vi "NP_Logging.vi"(0 "Instrument Channel":string="GPIB/0:4,0", 1 "Prefix (Instrument name)":string, 2 "String 1 Enable (T)":bool=TRUE, 3 "Generic Strings":bool, 5 "String 1 {Write} (in)":string, 7 "String 2 {Read} (in)":string, 9 "Filename (Data.log)":string="Data.log", 11 "error in (no error)":errorcluster, 12 "Operating Mode (Logging)":T1=enum."Logging", 13 "String 2 Enable (T)":bool=TRUE) -> (4 "Instrument Channel out":string="GPIB/0:4,0", 6 "String 1 {Write} (out)":string, 8 "String 2 {Read} (out)":string, 15 "error out":errorcluster)   [LabVIEW 2013]
doc: "This VI will enable logging of communication to a text file.\n\nIt will put timestamp and strings in the log file. \n\nIt can be used for Query/Response, or Generically for any logging.\nThe Label will be after the timestamp.\n\nNormal Operating Mode will disable logging."
uses:
  ctl_OperatingMode.ctl
panel:
  out "Target path":path
  in  "Show Interval":bool
  # "If Generic then Prefix will not indicate Write and Response."
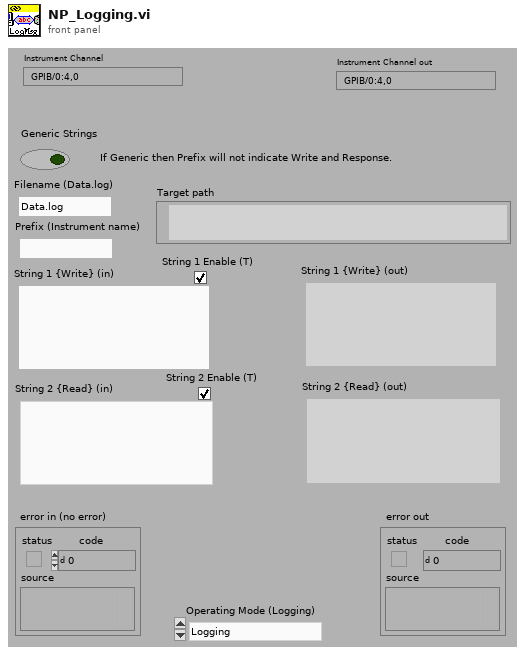
[diagram p1: front panel]
types:
  T1 = typedef "ctl_OperatingMode.ctl" = enum16{"Normal", "Logging", "Simulation w/Zeroes", "Simulation from Log File"}
  T2 = enum32{"invalid app kind", "Development System", "Run Time System", "Student Edition", "Embedded LabVIEW", "Evaluation", "Custom"}
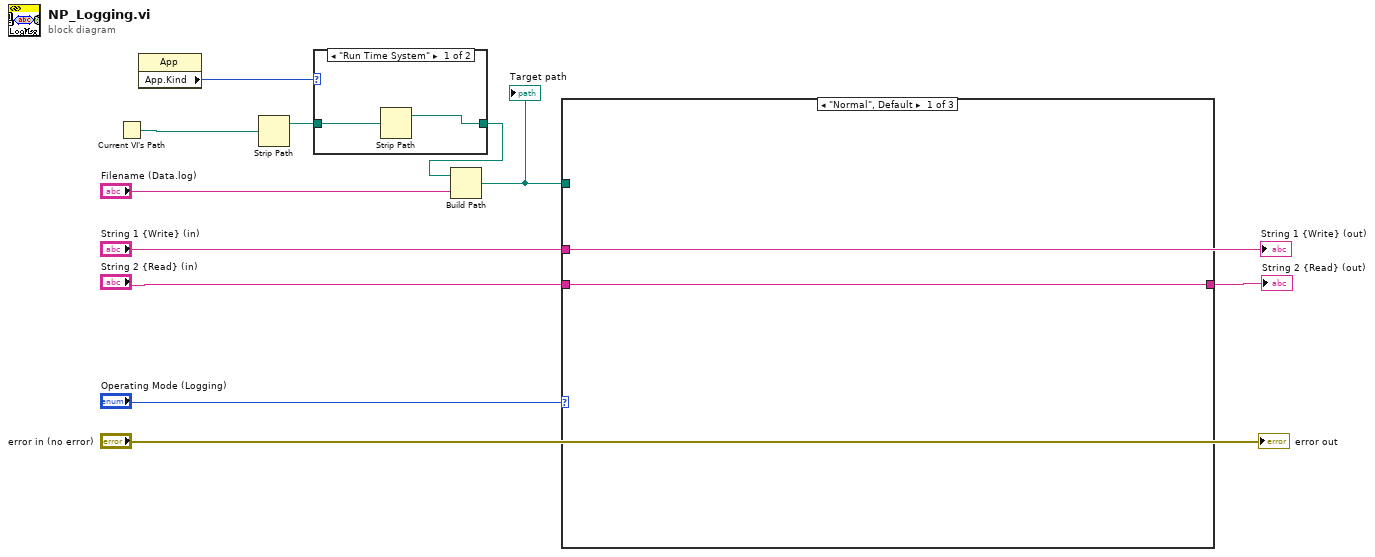
[diagram p0: block diagram]
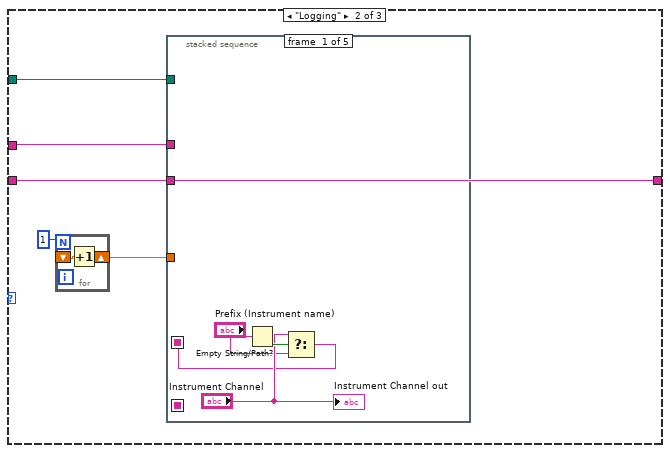
[diagram p3: hidden frame]
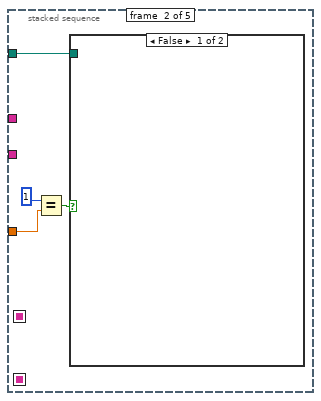
[diagram p4: hidden frame]
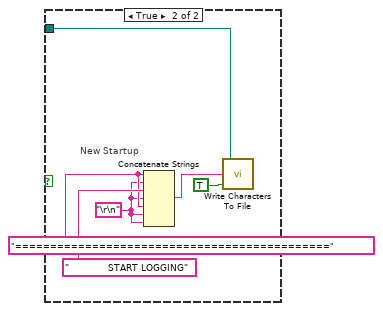
[diagram p5: hidden frame]
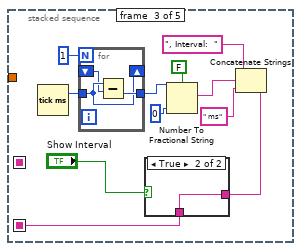
[diagram p6: hidden frame]
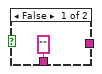
[diagram p7: hidden frame]
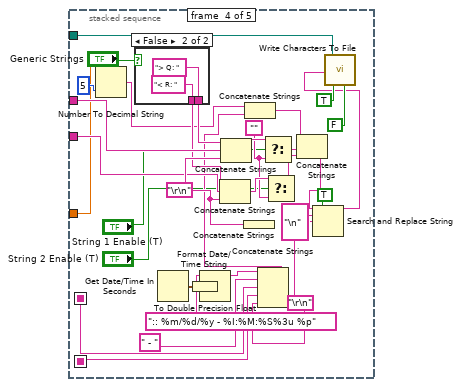
[diagram p8: hidden frame]
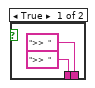
[diagram p9: hidden frame]
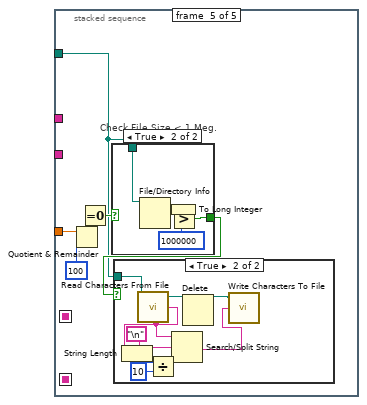
[diagram p10: hidden frame]
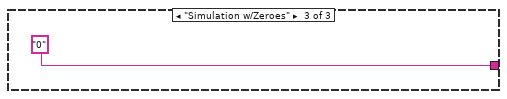
[diagram p13: hidden frame]
diagram:
  n1 = Current VI's Path() -> (path=w2:path)
  n2 = property class="App"() -> ("App.Kind"=w4:T2)  [unwired: 2 in, 2 out]
  n3 = Strip Path(path=w2) -> (stripped path=w3:path)  [unwired: 1 out]
  n4 = case shown="\"Run Time System\"" w4 {
    tunnel: w3 -> [w13 w14]
    tunnel: [w12 w14] -> w1
    frame "Run Time System" {
      n5 = Strip Path(path=w13) -> (stripped path=w12:path)  [unwired: 1 out]
    }
    frame Default {
    }
  }
  n6 = Build Path(base path=w1, name or relative path="Filename (Data.log)") -> (appended path=w5:path)
  "Target path" <- w5
  n7 = case shown="\"Normal\", Default" "Operating Mode (Logging)" {
    tunnel: "String 1 {Write} (in)" -> [_ w19 _]
    tunnel: "String 2 {Read} (in)" -> [w15 w20 _]
    tunnel: [w15 w20 "0"] -> w10
    tunnel: w5 -> [_ w18 _]
    frame "Normal", Default {
    }
    frame "Logging" {
      n8 = for {
        N: 1 -> [_]
        shift-right: [w21] -> w17
        shift-left: _ -> [w22]
        n9 = Increment(x=w22) -> (x+1=w21:dbl)
      }
      n10 = stacked-sequence {
        seq-local: [w23 _ _ _ _] -> [_ _ _ w62 _]
        seq-local: [_ _ w37 _ _] -> [_ _ _ w57 _]
        tunnel: w20 -> [_ _ _ w76 _]
        tunnel: w19 -> [_ _ _ w83 _]
        tunnel: w18 -> [_ w28 _ w54 w91]
        tunnel: w17 -> [_ w27 _ w53 w90]
        frame #0 {
          n11 = Empty String/Path?(string/path="Prefix (Instrument name)") -> (empty?=w26:bool)
          n12 = Select(t="Instrument Channel", s=w26, f="Prefix (Instrument name)") -> (s? t:f=w23:string)
          "Instrument Channel out" <- "Instrument Channel"
        }
        frame #1 {
          n13 = Equal?(x=1, y=w27) -> (x = y?=w29:bool)
          n14 = case shown="False" w29 {
            tunnel: w28 -> [_ w31]
            frame False {
            }
            frame True {
              w33 = "\r\n"
              w34 = "============================================="
              # "New Startup"
              n15 = Concatenate Strings(w34, w33, "             START LOGGING", w33, w34, w33, w33) -> (w32:string)
              n16 = call <vilib>:"Write Characters To File.vi"("append to file? (new file:F)"=TRUE, "character string"=w32, "file path (dialog if empty)"=w31) -> ()  [unwired: 2 in, 1 out]
            }
          }
        }
        frame #2 {
          n17 = Tick Count (ms)() -> (millisecond timer value=w47:u32)
          n18 = for {
            N: 1 -> [_]
            shift-right: [w51] -> _
            shift-left: _ -> [w50]
            tunnel: w47 -> [w51]
            tunnel: [w52] -> w45
            n19 = Subtract(x=w51, y=w50) -> (x-y=w52:u32)
          }
          n20 = Number To Fractional String(use system decimal point (T)=FALSE, number=w45, precision (6)=i16 0) -> (F-format string=w42:string)  [unwired: 1 in]
          n21 = Concatenate Strings(", Interval:  ", w42, " ms") -> (w38:string)
          n22 = case shown="True" "Show Interval" {
            tunnel: w38 -> [_ w49]
            tunnel: ["" w49] -> w37
            frame False {
            }
            frame True {
            }
          }
        }
        frame #3 {
          w67 = ""
          w77 = "\r\n"
          w56 = "\r\n"
          n23 = Number To Decimal String(number=w53, width (-)=i16 5) -> (decimal integer string=w74:string)
          n24 = case shown="False" "Generic Strings" {
            tunnel: [">>  " "< R: "] -> w75
            tunnel: [">>  " "> Q: "] -> w79
            frame True {
            }
            frame False {
            }
          }
          n25 = Get Date/Time In Seconds() -> (seconds since 1Jan1904=w55:timestamp)
          n26 = To Double Precision Float(number=w55) -> (double precision float=w82:dbl)
          n27 = Format Date/Time String(time format string (%c)=":: %m/%d/%y - %I:%M:%S%3u %p", seconds (now)=w82) -> (date/time string=w64:string)  [unwired: 1 in]
          n28 = Concatenate Strings(w75, w76, w77) -> (w71:string)
          n29 = Concatenate Strings(w79, w83, w77) -> (w69:string)
          n30 = Concatenate Strings(w77) -> ()  [unwired: 1 out]
          n31 = Concatenate Strings(w64, " - ", w62, w57, w56) -> (w73:string)
          n32 = Concatenate Strings(w74, w73) -> (w72:string)
          n33 = Select(t=w69, s="String 1 Enable (T)", f=w67) -> (s? t:f=w70:string)
          n34 = Select(t=w71, s="String 2 Enable (T)", f=w67) -> (s? t:f=w68:string)
          n35 = Concatenate Strings(w72, w70, w68) -> (w61:string)
          n36 = Search and Replace String(replace all?=TRUE ("replace all? (F)"), input string=w61, search string="\n", replace string=w56) -> (result string=w58:string)  [unwired: 4 in, 3 out]
          n37 = call <vilib>:"Write Characters To File.vi"("convert eol? (no:F)"=FALSE, "append to file? (new file:F)"=TRUE, "character string"=w58, "file path (dialog if empty)"=w54) -> ()  [unwired: 1 in, 1 out]
        }
        frame #4 {
          # "Check File Size < 1 Meg."
          n38 = Quotient & Remainder(x=w90, y=100) -> (x-y*floor(x/y)=w94:i32)  [unwired: 1 out]
          n39 = Equal To 0?(x=w94) -> (x = 0?=w93:bool)
          n40 = case shown="True" w93 {
            selector: w93 -> [w105 _]
            tunnel: w91 -> [_ w110]
            tunnel: [w105 w107] -> w92
            frame False {
            }
            frame True {
              n41 = File/Directory Info(path=w110) -> (size=w106:i64)  [unwired: 1 in, 6 out]
              n42 = To Long Integer(number=w106) -> (32bit integer=w109:i32)
              n43 = Greater?(x=w109, y=1000000) -> (0:w107:bool)
            }
          }
          n44 = case shown="True" w92 {
            tunnel: w91 -> [_ w104]
            frame False {
            }
            frame True {
              n45 = call <vilib>:"Read Characters From File.vi"("file path (dialog if empty)"=w104) -> ("new file path (NotAPath if cancelled)"=w97:path, "character string"=w102:string)  [unwired: 5 in, 2 out]
              n46 = String Length(string=w102) -> (length=w101:i32)
              n47 = Divide(x=w101, y=10) -> (x/y=w99:dbl)
              n48 = Search/Split String(string=w102, search string/char (-)="\n", offset (0)=w99) -> (match + rest of string=w98:string)  [unwired: 2 out]
              n49 = Delete(path (use dialog)=w97) -> (deleted path=w96:path)  [unwired: 4 in, 2 out]
              n50 = call <vilib>:"Write Characters To File.vi"("character string"=w98, "file path (dialog if empty)"=w96) -> ()  [unwired: 3 in, 1 out]
            }
          }
        }
      }
    }
    frame "Simulation w/Zeroes" {
    }
  }
  "String 2 {Read} (out)" <- w10
  "error out" <- "error in (no error)"
  "String 1 {Write} (out)" <- "String 1 {Write} (in)"
